vi "加线.vi"(0 "质心X":sgl, 1 "是否加线":bool, 5 "质心X 2":sgl, 7 "Image in":T1, 9 "质心Y":sgl, 11 "质心Y 2":sgl, 12 "Color":u32(colorbox)=16711680) -> (4 "Image Out 2":T1)   [LabVIEW 2015]
uses:
  <vilib>/vision/Image Controls.llb/IMAQ Image.ctl
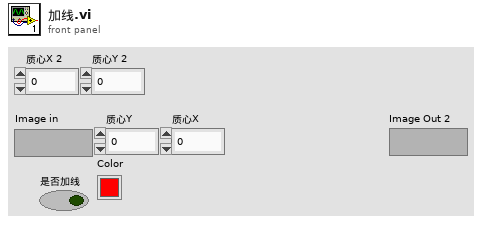
[diagram p1: front panel]
types:
  T1 = typedef "IMAQ Image.ctl" = refnum<image>
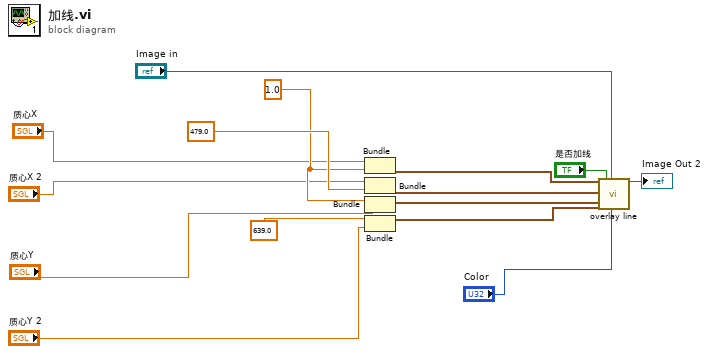
[diagram p0: block diagram]
diagram:
  w8 = sgl 1.0 ("element")
  n1 = Bundle("质心X"="质心X", "element"=w8) -> (w14:cluster{"质心X":sgl, "element":sgl})  [unwired: 1 in]
  n2 = Bundle("质心X 2"="质心X 2", "element"=sgl 479.0) -> (w13:cluster{"质心X 2":sgl, "element":sgl})  [unwired: 1 in]
  n3 = Bundle("element"=w8, "质心Y"="质心Y") -> (w12:cluster{"element":sgl, "质心Y":sgl})  [unwired: 1 in]
  n4 = Bundle("element"=sgl 639.0, "质心Y 2"="质心Y 2") -> (w11:cluster{"element":sgl, "质心Y 2":sgl})  [unwired: 1 in]
  n5 = call "overlay line.vi"("垂直方向第一点"=w14, "垂直方向第二点"=w13, "水平方向第一点"=w12, "水平方向第二点"=w11, "触发"="是否加线", "Image in"="Image in", "Color"="Color") -> ("Image Out 2"=→"Image Out 2":T1)  [unwired: 11 in, 1 out]
